vi "Configure Supply.vi"(0 "Supply Handle in":refnum<k15>, 1 "Channel Name(s)":string, 5 "Supply Configuration":T1={"output function"=1006, "Voltage Level (V)"=3.0, "Current Level (A)"=0.001, "Voltage Limit (V)"=1.0, "Current Limit (A)"=0.001, "Transient Response Mode"=1038, "Custom Transient Config"={"Gain Bandwidth"=5000.0, "Compensation Frequency"=50000.0, "Pole Zero Ratio"=1.0}} {"Transient Response Mode" items=["Slow"=1041, "Normal"=1038, "Fast"=1039, "Custom"=1042]; "output function" items=["DC Voltage"=1006, "DC Current"=1007, "Pulse Voltage"=1049, "Pulse Current"=1050]}, 11 "error in (no error)":errorcluster) -> (4 "Supply Handle out":refnum<k15>, 15 "error out":errorcluster)   [LabVIEW 2016, in "Supply.lvlib"]
uses:
  Supply.lvlib
  Typedefs/Supply Configuration.ctl
  <instrlib>/niDCPower/nidcpower.llb/niDCPower Output Function.ctl
  Typedefs/Custom Transient Response.ctl
  <instrlib>/niDCPower/nidcpower.llb/niDCPower Source Mode.ctl
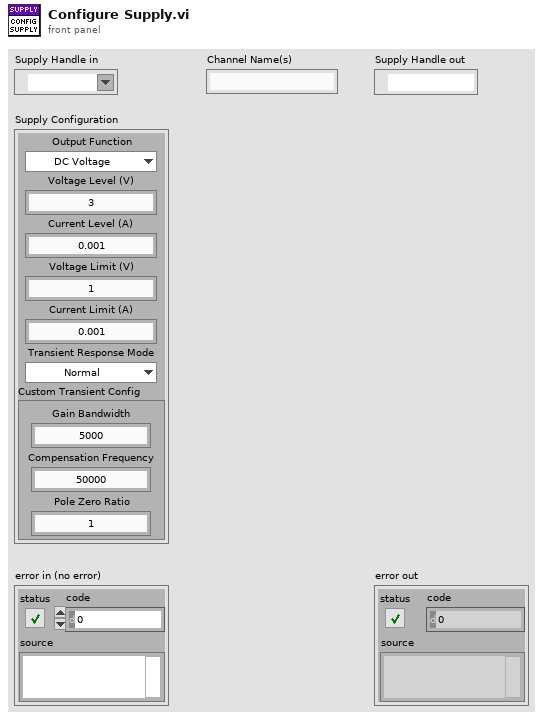
[diagram p1: front panel]
types:
  T1 = typedef "Supply.lvlib/Supply Configuration.ctl" = cluster{"output function":T2, "Voltage Level (V)":dbl, "Current Level (A)":dbl, "Voltage Limit (V)":dbl, "Current Limit (A)":dbl, "Transient Response Mode":i32, "Custom Transient Config":T3}
  T2 = typedef "niDCPower Output Function.ctl" = i32
  T3 = typedef "Supply.lvlib/Custom Transient Response.ctl" = cluster{"Gain Bandwidth":dbl, "Compensation Frequency":dbl, "Pole Zero Ratio":dbl}
  T4 = typedef "niDCPower Source Mode.ctl" = i32
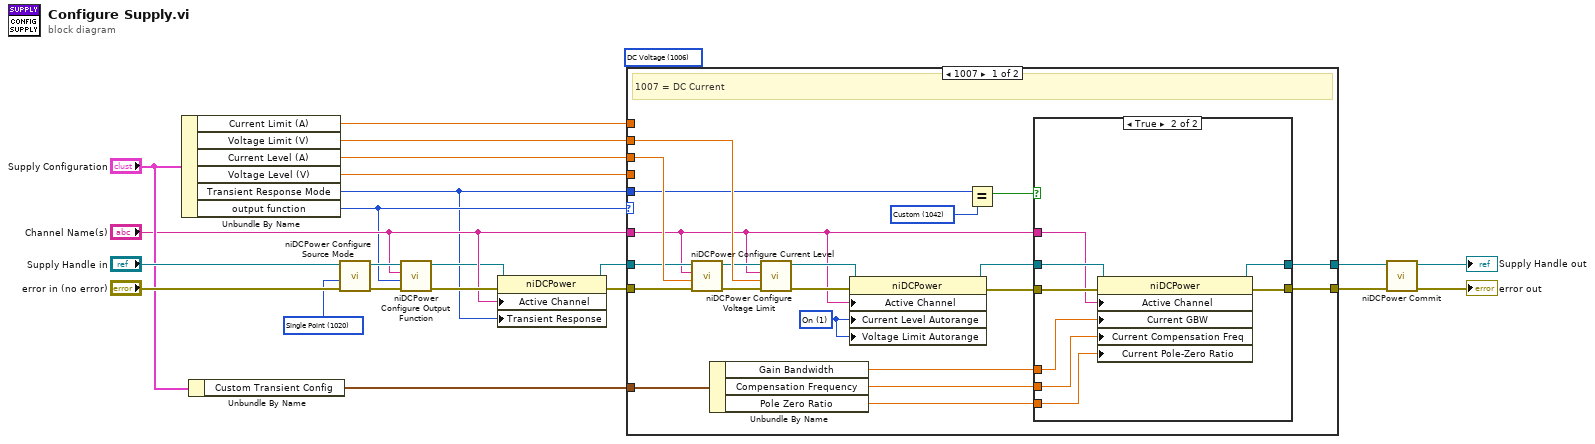
[diagram p0: block diagram]
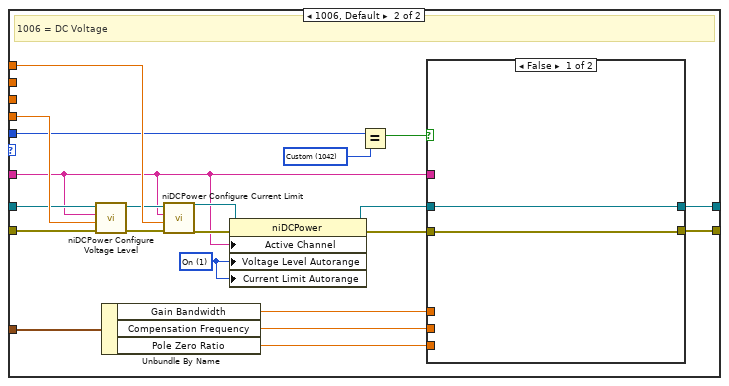
[diagram p3: hidden frame]
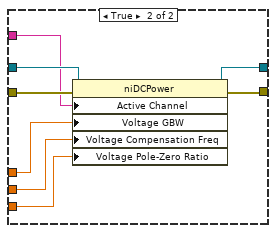
[diagram p4: hidden frame]
diagram:
  (unwired) T2 1006 items=["DC Voltage"=1006, "DC Current"=1007, "Pulse Voltage"=1049, "Pulse Current"=1050] ("Output Function")
  w16 = T4 1020 items=["Single Point"=1020, "Sequence"=1021] ("source mode")
  n1 = Unbundle By Name("Supply Configuration") -> ("Current Limit (A)"=w13:dbl, "Voltage Limit (V)"=w12:dbl, "Current Level (A)"=w14:dbl, "Voltage Level (V)"=w15:dbl, "Transient Response Mode"=w2:i32, "output function"=w3:T2)
  n2 = Unbundle By Name("Supply Configuration") -> ("Custom Transient Config"=w1:T3)
  n3 = call <instrlib>:"niDCPower Configure Source Mode.vi"("error in (no error)"="error in (no error)", "source mode"=w16, "instrument handle"="Supply Handle in") -> ("error out"=w22:errorcluster, "instrument handle out"=w10:refnum<k15>)  [unwired: 7 out]
  n4 = call <instrlib>:"niDCPower Configure Output Function.vi"("error in (no error)"=w22, "output function"=w3, "channel name"="Channel Name(s)", "instrument handle"=w10) -> ("error out"=w17:errorcluster, "instrument handle out"=w5:refnum<k15>)  [unwired: 6 in]
  n5 = property class="niDCPower"(reference=w5, error in=w17, "Active Channel"="Channel Name(s)", "Transient Response"=w2) -> (reference out=w4:refnum<k15>, error out=w18:errorcluster)
  n6 = case shown="1007" w3 {
    tunnel: [w31 w63] -> w9
    tunnel: "Channel Name(s)" -> [w24 w58]
    tunnel: w15 -> [_ w69]
    tunnel: w14 -> [w38 _]
    tunnel: w13 -> [_ w68]
    tunnel: w12 -> [w37 _]
    tunnel: [w41 w71] -> w20
    tunnel: w4 -> [w34 w65]
    tunnel: w18 -> [w42 w73]
    tunnel: w2 -> [w23 w62]
    tunnel: w1 -> [w30 w57]
    frame 1007 {
      w33 = 1042 items=["Slow"=1041, "Normal"=1038, "Fast"=1039, "Custom"=1042] ("Source:Transient Response")
      w35 = 1 items=["Off", "On"] ("Source:DC Voltage:Voltage Level Autorange")
      # "1007 = DC Current"
      n7 = call <instrlib>:"niDCPower Configure Current Level.vi"("error in (no error)"=w42, "current level"=w38, "channel name"=w24, "instrument handle"=w34) -> ("error out"=w43:errorcluster, "instrument handle out"=w36:refnum<k15>)  [unwired: 6 in]
      n8 = Unbundle By Name(w30) -> ("Gain Bandwidth"=w29:dbl, "Compensation Frequency"=w28:dbl, "Pole Zero Ratio"=w27:dbl)
      n9 = call <instrlib>:"niDCPower Configure Voltage Limit.vi"("error in (no error)"=w43, "voltage limit"=w37, "channel name"=w24, "instrument handle"=w36) -> ("error out"=w39:errorcluster, "instrument handle out"=w26:refnum<k15>)  [unwired: 6 in]
      n10 = property class="niDCPower"(reference=w26, error in=w39, "Active Channel"=w24, "Current Level Autorange"=w35, "Voltage Limit Autorange"=w35) -> (reference out=w25:refnum<k15>, error out=w40:errorcluster)
      n11 = Equal?(x=w23, y=w33) -> (x = y?=w32:bool)
      n12 = case shown="True" w32 {
        tunnel: [w45 w53] -> w41
        tunnel: [w44 w51] -> w31
        tunnel: w40 -> [w45 w52]
        tunnel: w25 -> [w44 w50]
        tunnel: w24 -> [_ w49]
        tunnel: w29 -> [_ w48]
        tunnel: w28 -> [_ w47]
        tunnel: w27 -> [_ w46]
        frame False {
        }
        frame True {
          n13 = property class="niDCPower"(reference=w50, error in=w52, "Active Channel"=w49, "Current GBW"=w48, "Current Compensation Freq"=w47, "Current Pole-Zero Ratio"=w46) -> (reference out=w51:refnum<k15>, error out=w53:errorcluster)
        }
      }
    }
    frame 1006, Default {
      w61 = 1042 items=["Slow"=1041, "Normal"=1038, "Fast"=1039, "Custom"=1042] ("Source:Transient Response")
      w66 = 1 items=["Off", "On"] ("Source:DC Voltage:Voltage Level Autorange")
      # "1006 = DC Voltage"
      n14 = call <instrlib>:"niDCPower Configure Voltage Level.vi"("error in (no error)"=w73, "voltage level"=w69, "channel name"=w58, "instrument handle"=w65) -> ("error out"=w74:errorcluster, "instrument handle out"=w67:refnum<k15>)  [unwired: 6 out]
      n15 = Unbundle By Name(w57) -> ("Gain Bandwidth"=w56:dbl, "Compensation Frequency"=w55:dbl, "Pole Zero Ratio"=w54:dbl)
      n16 = call <instrlib>:"niDCPower Configure Current Limit.vi"("error in (no error)"=w74, "current limit"=w68, "channel name"=w58, "instrument handle"=w67) -> ("error out"=w72:errorcluster, "instrument handle out"=w64:refnum<k15>)  [unwired: 1 in, 5 out]
      n17 = property class="niDCPower"(reference=w64, error in=w72, "Active Channel"=w58, "Voltage Level Autorange"=w66, "Current Limit Autorange"=w66) -> (reference out=w59:refnum<k15>, error out=w70:errorcluster)
      n18 = Equal?(x=w62, y=w61) -> (x = y?=w60:bool)
      n19 = case shown="False" w60 {
        tunnel: [w76 w84] -> w71
        tunnel: [w75 w82] -> w63
        tunnel: w70 -> [w76 w83]
        tunnel: w59 -> [w75 w81]
        tunnel: w58 -> [_ w80]
        tunnel: w56 -> [_ w79]
        tunnel: w55 -> [_ w78]
        tunnel: w54 -> [_ w77]
        frame False {
        }
        frame True {
          n20 = property class="niDCPower"(reference=w81, error in=w83, "Active Channel"=w80, "Voltage GBW"=w79, "Voltage Compensation Freq"=w78, "Voltage Pole-Zero Ratio"=w77) -> (reference out=w82:refnum<k15>, error out=w84:errorcluster)
        }
      }
    }
  }
  n21 = call <instrlib>:"niDCPower Commit.vi"("error in (no error)"=w20, "instrument handle"=w9) -> ("error out"=→"error out":errorcluster, "instrument handle out"=→"Supply Handle out":refnum<k15>)  [unwired: 8 in]
